vi "2P_AdapUprite_Linlin.vi"() -> ()   [LabVIEW 2015] (continued)
                                n3537 = call "waveformparamsv2.vi"("command"="add AO", "add AO"=w248) -> ()  [unwired: 3 in, 3 out]
                              }
                              frame "Matlab" {
                                w274 = 0.0 ("Repeats")
                                n3538 = local read "Meastab"() -> (w270:enum32{"X-Y Image", "Linescan", "Timetrace"})
                                n3539 = call "waveformparamsv2.vi"("command"="get") -> ("Params out"=w281:T17)  [unwired: 4 in, 2 out]
                                n3540 = Unbundle By Name(w281) -> ("AO parameters"=w278:T18)
                                n3541 = case shown="\"Timetrace\"" w270 {
                                tunnel: [w284 w285] -> w269
                                frame "X-Y Image", Default {
                                n3542 = local read "Sampling rate"() -> (w284:dbl)
                                }
                                frame "Timetrace" {
                                n3543 = local read "srateAODOtt"() -> (w285:dbl)
                                }
                                }
                                n3544 = local read "Matlab waveform path"() -> (w271:path)
                                n3545 = local read "Matlab padding value"() -> (w273:dbl)
                                n3546 = Index Array(array=w278, index=0) -> (element=w279:T19)
                                n3547 = call "matlabwfexistsdialogue.vi"("Matlab waveform path"=w271) -> ("mtalab waveform path out"=w272:path)
                                n3548 = Bundle By Name(cluster=w279, "AOtab"=2.0 ("Repeats"), "Repeats"=w274, "Cycles"=w274, "Start amplitude (V)"=w274, "Baseline (V)"=w274, "Step size (V)"=w274, "DC (%)"=w274, "Sampling frequency (Hz)"=w269, "Period (ms)"=w274, "Offset (V)"=w274, "Amplitude (V)"=w274, "Frequency"=w274, "Tri Repeats"=w274, "phase shift (ms)"=w274, "Pulses"=w274, "Matlab wave file"=w272, "padding value"=w273) -> (w276:T19)
                                n3549 = Build Array(w276) -> (w275:T18)
                                n3550 = call "waveformparamsv2.vi"("command"="add AO", "add AO"=w275) -> ()  [unwired: 3 in, 3 out]
                              }
                              frame "Triangle" {
                                w291 = 0.0 ("Offset (V)")
                                n3551 = local read "Meastab"() -> (w287:enum32{"X-Y Image", "Linescan", "Timetrace"})
                                n3552 = call "waveformparamsv2.vi"("command"="get") -> ("Params out"=w303:T17)  [unwired: 4 in, 2 out]
                                n3553 = Unbundle By Name(w303) -> ("AO parameters"=w300:T18)
                                n3554 = case shown="\"Timetrace\"" w287 {
                                tunnel: [w305 w306] -> w286
                                frame "X-Y Image", Default {
                                n3555 = local read "Sampling rate"() -> (w305:dbl)
                                }
                                frame "Timetrace" {
                                n3556 = local read "srateAODOtt"() -> (w306:dbl)
                                }
                                }
                                n3557 = local read "Tri padding value"() -> (w289:dbl)
                                n3558 = local read "Amplitude (V)"() -> (w294:dbl)
                                n3559 = local read "Tri Phase (s)"() -> (w290:dbl)
                                n3560 = local read "Tri Repeats"() -> (w292:dbl)
                                n3561 = local read "Frequency"() -> (w293:dbl)
                                n3562 = local read "Offset (V)"() -> (w295:dbl)
                                n3563 = Index Array(array=w300, index=0) -> (element=w301:T19)
                                n3564 = Bundle By Name(cluster=w301, "AOtab"=1.0 ("Repeats"), "Repeats"=w291, "Cycles"=w291, "Start amplitude (V)"=w291, "Baseline (V)"=w291, "Step size (V)"=w291, "DC (%)"=w291, "Sampling frequency (Hz)"=w286, "Period (ms)"=w291, "Offset (V)"=w295, "Amplitude (V)"=w294, "Frequency"=w293, "Tri Repeats"=w292, "phase shift (ms)"=w291, "Pulses"=w291, "Matlab wave file"=path "", "Tri phase"=w290, "padding value"=w289) -> (w298:T19)
                                n3565 = Build Array(w298) -> (w297:T18)
                                n3566 = call "waveformparamsv2.vi"("command"="add AO", "add AO"=w297) -> ()  [unwired: 3 in, 3 out]
                              }
                            }
                          }
                        }
                      }
                    }
                  }
                  frame #6 {
                    n3567 = case shown="True" w307 {
                      frame False {
                      }
                      frame True {
                        n3568 = local read "addAO"() -> (w308:bool)
                        n3569 = case shown="True" w308 {
                          frame False {
                          }
                          frame True {
                            # "add waveform to waveform array; correct waveform lengths and plot"
                            n3570 = local read "Meastab"() -> (w312:enum32{"X-Y Image", "Linescan", "Timetrace"})
                            n3571 = local read "Build analog waveform tabs"() -> (w322:enum32{"Square", "Triangle", "Matlab"})
                            n3572 = case shown="\"Timetrace\"" w312 {
                              tunnel: [w330 w331] -> w311
                              frame "X-Y Image", Default {
                                n3573 = local read "Sampling rate"() -> (w330:dbl)
                              }
                              frame "Timetrace" {
                                n3574 = local read "srateAODOtt"() -> (w331:dbl)
                              }
                            }
                            n3575 = call "waveformparamsv2.vi"("command"="get last AO") -> ("last AO"=w324:T19)  [unwired: 4 in, 2 out]
                            n3576 = case shown="\"Square\", Default" w322 {
                              tunnel: w324 -> [w334 w336 w338]
                              tunnel: [w333 w335 w337] -> w323
                              frame "Square", Default {
                                n3577 = call "generateRampedSquareWave_fromAOparameters.vi"("AO params"=w334) -> ("Waveform"=w333:waveform(dbl))  [unwired: 1 out]
                              }
                              frame "Triangle" {
                                n3578 = call "generateTriWave_fromAOparameters.vi"("AO params"=w336) -> ("Waveform"=w335:waveform(dbl))  [unwired: 1 out]
                              }
                              frame "Matlab" {
                                n3579 = call "matlabAOwffromparam.vi"("Cluster"=w338) -> ("Waveform"=w337:waveform(dbl))  [unwired: 1 out]
                              }
                            }
                            n3580 = property on="refwf" class="Ring (strict)"() -> ("RingText.Text"=w315:string)  [unwired: 2 in, 2 out]
                            n3581 = call "waveformsAObuffer.vi"("command"="get") -> ("AO wf out"=w328:waveform(dbl)[])  [unwired: 1 in]
                            n3582 = Build Array (concatenate)(w328, w323) -> (w325:waveform(dbl)[])
                            n3583 = call "waveformsDObuffer.vi"("command"="get") -> ("DO wf out"=w320:digitalwaveform[])  [unwired: 1 in]
                            n3584 = call "correctwaveformsizetemp.vi"("new sampling frequency (Hz)"=w311, "start"=FALSE, "reference waveforms to"=w315, "Analog waveforms in"=w325, "stop"=FALSE, "Digital waveforms in"=w320) -> ("analog wf out"=w318:waveform(dbl)[], "Digital wf out"=w316:digitalwaveform[], "measpoints"=w313:i32)
                            n3585 = local write "Analog Lines Plot"(w318) -> ()
                            n3586 = call "GetNumCamFramesv2.vi"("Digital Waveform Graph"=w316) -> ("Numeric"=w317:i32)  [unwired: 10 in]
                            n3587 = local write "Digital Lines Plot"(w316) -> ()
                            n3588 = call "waveformsAObuffer.vi"("AO wf in"=w318, "command"="set") -> ()  [unwired: 1 out]
                            n3589 = call "waveformsDObuffer.vi"("DO wf in"=w316, "command"="set") -> ()  [unwired: 1 out]
                            n3590 = local write "Total Camera Frames"(w317) -> ()
                            n3591 = local read "wavdet"() -> (w314:bool)
                            n3592 = case shown="True" w314 {
                              tunnel: w313 -> [_ w332]
                              frame False {
                              }
                              frame True {
                                n3593 = local write "# of frames"(w332) -> ()
                              }
                            }
                          }
                        }
                      }
                    }
                  }
                  frame #7 {
                    w340 = FALSE ("addAO")
                    # "set signaling boolean to false"
                    n3594 = case shown="True" w339 {
                      frame False {
                      }
                      frame True {
                        n3595 = local read "Build analog waveform tabs"() -> (w348:enum32{"Square", "Triangle", "Matlab"})
                        n3596 = case shown="\"Triangle\"" w348 {
                          frame "Square", Default {
                            n3597 = local write "not loaded"(FALSE ("not loaded")) -> ()
                          }
                          frame "Triangle" {
                            n3598 = local write "not loadedtri"(FALSE ("not loadedtri")) -> ()
                          }
                          frame "Matlab" {
                            n3599 = local write "not loadedml"(FALSE ("not loadedml")) -> ()
                          }
                        }
                      }
                    }
                    n3600 = local read "finite samples"() -> (w341:bool)
                    n3601 = local read "continuous"() -> (w342:bool)
                    n3602 = local read "wavdet"() -> (w343:bool)
                    n3603 = call "2pparameters.vi"("command"="get") -> ("params out"=w346:T12)  [unwired: 1 in]
                    n3604 = Bundle By Name(cluster=w346, "finite"=w341, "cont"=w342, "wavdet"=w343) -> (w344:T12)
                    n3605 = local write "addAO"(w340) -> ()
                    n3606 = property on="Add AO wave" class="Bool (strict)"("Val(Sgnl)"=w340) -> ()  [unwired: 2 in, 2 out]
                    n3607 = call "2pparameters.vi"("Params in"=w344, "command"="set") -> ()  [unwired: 1 out]
                  }
                }
              }
            }
          }
          event "AO channels": Value Change {
            n3608 = event-data() -> ()  [unwired: 1 in, 6 out]
            n3609 = local read "AO channels"() -> (w352:u32)
            n3610 = call "2pparameters.vi"("command"="get") -> ("params out"=w354:T12)  [unwired: 1 in]
            n3611 = Unbundle By Name(w354) -> ("aAO"=w353:u32[])
            n3612 = Search 1D Array(1D array=w353, element=w352) -> (index of element=w356:i32)  [unwired: 1 in]
            n3613 = Equal?(x=w356, y=-1.0) -> (x = y?=w357:bool)
            n3614 = case shown="False" w357 {
              tunnel: w356 -> [w359 _]
              frame False {
                n3615 = call "waveformparamsv2.vi"("command"="get") -> ("Params out"=w366:T17)  [unwired: 4 in, 2 out]
                n3616 = Unbundle By Name(w366) -> ("AO parameters"=w365:T18)
                n3617 = Index Array(array=w365, index=w359) -> (element=w382:T19)
                n3618 = Unbundle By Name(w382) -> ("AOtab"=w363:dbl, "Repeats"=w381:dbl, "Cycles"=w380:dbl, "Start amplitude (V)"=w379:dbl, "Baseline (V)"=w378:dbl, "Step size (V)"=w377:dbl, "DC (%)"=w376:dbl, "Sampling frequency (Hz)"=w375:dbl, "Period (ms)"=w374:dbl, "Offset (V)"=w373:dbl, "Amplitude (V)"=w372:dbl, "Frequency"=w371:dbl, "Tri Repeats"=w370:dbl, "phase shift (ms)"=w369:dbl, "Pulses"=w368:dbl, "Tri phase"=w364:dbl, "padding value"=w360:dbl, "Matlab wave file"=w361:path)
                n3619 = To Unsigned Long Integer(number=w363) -> (unsigned 32bit integer=w362:u32)
                n3620 = local write "Build analog waveform tabs"(w362) -> ()
                n3621 = local write "Matlab waveform path"(w361) -> ()
                n3622 = local write "phase shift (ms)"(w369) -> ()
                n3623 = local write "Repeats"(w381) -> ()
                n3624 = local write "Cycles"(w380) -> ()
                n3625 = local write "Amplitude (V)"(w372) -> ()
                n3626 = local write "Matlab padding value"(w360) -> ()
                n3627 = local write "Tri padding value"(w360) -> ()
                n3628 = local write "Start amplitude (V)"(w379) -> ()
                n3629 = local write "Tri Phase (s)"(w364) -> ()
                n3630 = local write "Period (ms)"(w374) -> ()
                n3631 = local write "Tri Repeats"(w370) -> ()
                n3632 = local write "Offset (V)"(w373) -> ()
                n3633 = local write "Frequency"(w371) -> ()
                n3634 = local write "Pulses"(w368) -> ()
                n3635 = local write "padding value"(w360) -> ()
                n3636 = local write "Sampling rate \ncurrent wf"(w375) -> ()
                n3637 = local write "Baseline (V)"(w378) -> ()
                n3638 = local write "Step size (V)"(w377) -> ()
                n3639 = local write "DC (%)"(w376) -> ()
              }
              frame True {
              }
            }
          }
          event "Rem AO wave": Value Change {
            n3640 = event-data() -> ("NewVal"=w383:bool)  [unwired: 1 in, 5 out]
            n3641 = case shown="True" w383 {
              frame False {
              }
              frame True {
                n3642 = stacked-sequence {
                  seq-local: [_ _ w489 _ _ _ _] -> [_ _ _ _ w509 w512 _]
                  frame #0 {
                    n3643 = local read "Measurement"() -> (w384:T4)
                    n3644 = case shown="\"Lifetime (contour)\"" w384 {
                      frame "X-Y-t movie", Default {
                        n3645 = local read "avpp"() -> (w405:i32)
                        n3646 = local read "Angle ref"() -> (w404:dbl)
                        n3647 = local read "ROI Type"() -> (w403:u16)
                        n3648 = local read "xpixels ref"() -> (w400:i32)
                        n3649 = local read "Vx-min ref"() -> (w399:dbl)
                        n3650 = local read "Vx-max ref"() -> (w398:dbl)
                        n3651 = local read "ypixels ref"() -> (w396:i32)
                        n3652 = local read "Vy-min ref"() -> (w397:dbl)
                        n3653 = local read "Vy-max ref"() -> (w393:dbl)
                        n3654 = local read "Sampling rate"() -> (w387:dbl)
                        n3655 = local read "finite samples"() -> (w388:bool)
                        n3656 = local read "continuous"() -> (w391:bool)
                        n3657 = local read "wavdet"() -> (w392:bool)
                        n3658 = local read "# of frames"() -> (w390:i32)
                        n3659 = local read "maxbufferAI"() -> (w389:i32)
                        n3660 = local read "Override AI buffer"() -> (w385:bool)
                        n3661 = call "2pparameters.vi"("command"="get") -> ("params out"=w402:T12)  [unwired: 1 in]
                        n3662 = Bundle By Name(cluster=w402, "type"="X-Y-t movie", "avpp"=w405, "Angle Img"=w404, "Xpixels Img"=w400, "Vx-min Img"=w399, "VX-max Img"=w398, "Ypixels Img"=w396, "Vy-min Img"=w397, "Vy-max Img"=w393, "srate"=w387, "srate Img"=w387, "finite"=w388, "cont"=w391, "wavdet"=w392, "measpoints"=w390, "maxbufferAI"=w389, "Drawing Mode"=w403, "Vz-reset"=0.0, "AIoverride"=w385) -> (w394:T12)
                        n3663 = call "2pparameters.vi"("Params in"=w394, "command"="set") -> ()  [unwired: 1 out]
                      }
                      frame "X-Y-Z stack" {
                        n3664 = call "2pparameters.vi"("command"="get") -> ("params out"=w409:T12)  [unwired: 1 in]
                        n3665 = Bundle By Name(cluster=w409, "type"="X-Y-Z stack") -> (w407:T12)
                        n3666 = call "2pparameters.vi"("Params in"=w407, "command"="set") -> ()  [unwired: 1 out]
                      }
                      frame "Lifetime (scan)" {
                        n3667 = call "2pparameters.vi"("command"="get") -> ("params out"=w414:T12)  [unwired: 1 in]
                        n3668 = Bundle By Name(cluster=w414, "type"="Lifetime (scan)") -> (w412:T12)
                        n3669 = call "2pparameters.vi"("Params in"=w412, "command"="set") -> ()  [unwired: 1 out]
                      }
                      frame "Lifetime (contour)" {
                        n3670 = local read "Vy-min draw"() -> (w424:dbl)
                        n3671 = local read "Vy-max draw"() -> (w423:dbl)
                        n3672 = local read "Vx-min draw"() -> (w426:dbl)
                        n3673 = local read "Vx-max draw"() -> (w425:dbl)
                        n3674 = local read "xpixels ref"() -> (w422:i32)
                        n3675 = local read "ypixels ref"() -> (w421:i32)
                        n3676 = local read "ROI Type"() -> (w420:u16)
                        n3677 = local read "srateAODOtt"() -> (w431:dbl)
                        n3678 = local read "# of frames"() -> (w436:i32)
                        n3679 = local read "refreshtime"() -> (w428:dbl)
                        n3680 = local read "Pel"() -> (w419:dbl)
                        n3681 = local read "bin"() -> (w434:dbl)
                        n3682 = local read "Override AI buffer"() -> (w417:bool)
                        n3683 = local read "finite samples"() -> (w443:bool)
                        n3684 = local read "srateAODOtt"() -> (w430:dbl)
                        n3685 = local read "srateAODOtt"() -> (w437:dbl)
                        n3686 = local read "continuous"() -> (w442:bool)
                        n3687 = local read "Angle ref"() -> (w427:dbl)
                        n3688 = local read "wavdet"() -> (w444:bool)
                        n3689 = local read "Vx-ref"() -> (w439:dbl)
                        n3690 = local read "Vy-ref"() -> (w441:dbl)
                        n3691 = local read "avpp"() -> (w440:i32)
                        n3692 = call "tt_timeandsamples.vi"("bin"=w434, "refreshtime"=w428, "srateAODOtt"=w431, "tot#ofsamples"=w436) -> ("refreshrate"=w432:dbl, "refreshbuffer"=w433:i32, "timetracecycles"=w438:i32)  [unwired: 5 in]
                        n3693 = local read "bin"() -> (w435:dbl)
                        n3694 = call "2pparameters.vi"("command"="get") -> ("params out"=w447:T12)  [unwired: 1 in]
                        n3695 = Bundle By Name(cluster=w447, "Drawing Mode"=w420, "measpoints"=w436, "tt_cycles"=w438, "refreshbuffer"=w433, "refreshrate"=w432, "Vx-ref"=w439, "Vy-ref"=w441, "srate"=w430, "finite"=w443, "cont"=w442, "wavdet"=w444, "avpp"=w440, "srateAODO"=w437, "bufferAI"=w433, "bin"=w435, "Angle Img"=w427, "Vxminref"=w426, "Vxmaxref"=w425, "Vyminref"=w424, "Vymaxref"=w423, "Xpixels Img"=w422, "Ypixels Img"=w421, "Pel"=w419, "Vz-reset"=0.0, "AIoverride"=w417, "type"="Lifetime (contour)") -> (w445:T12)
                        n3696 = Reciprocal(x=w432) -> (1/x=w429:dbl)
                        n3697 = local write "refreshtime"(w429) -> ()
                        n3698 = call "2pparameters.vi"("Params in"=w445, "command"="set") -> ()  [unwired: 1 out]
                      }
                      frame "X-Y-Z-t movie" {
                      }
                      frame "linescan" {
                      }
                      frame "Timetrace" {
                        n3699 = local read "Vy-min draw"() -> (w457:dbl)
                        n3700 = local read "Vy-max draw"() -> (w456:dbl)
                        n3701 = local read "Vx-min draw"() -> (w459:dbl)
                        n3702 = local read "Vx-max draw"() -> (w458:dbl)
                        n3703 = local read "xpixels ref"() -> (w455:i32)
                        n3704 = local read "ypixels ref"() -> (w454:i32)
                        n3705 = local read "ROI Type"() -> (w453:u16)
                        n3706 = local read "srateAODOtt"() -> (w464:dbl)
                        n3707 = local read "# of frames"() -> (w469:i32)
                        n3708 = local read "refreshtime"() -> (w461:dbl)
                        n3709 = local read "Pel"() -> (w452:dbl)
                        n3710 = local read "bin"() -> (w467:dbl)
                        n3711 = local read "Override AI buffer"() -> (w450:bool)
                        n3712 = local read "finite samples"() -> (w476:bool)
                        n3713 = local read "srateAODOtt"() -> (w463:dbl)
                        n3714 = local read "srateAODOtt"() -> (w470:dbl)
                        n3715 = local read "continuous"() -> (w475:bool)
                        n3716 = local read "Angle ref"() -> (w460:dbl)
                        n3717 = local read "wavdet"() -> (w477:bool)
                        n3718 = local read "Vx-ref"() -> (w472:dbl)
                        n3719 = local read "Vy-ref"() -> (w474:dbl)
                        n3720 = local read "avpp"() -> (w473:i32)
                        n3721 = call "tt_timeandsamples.vi"("bin"=w467, "refreshtime"=w461, "srateAODOtt"=w464, "tot#ofsamples"=w469) -> ("refreshrate"=w465:dbl, "refreshbuffer"=w466:i32, "timetracecycles"=w471:i32)  [unwired: 5 in]
                        n3722 = local read "bin"() -> (w468:dbl)
                        n3723 = call "2pparameters.vi"("command"="get") -> ("params out"=w480:T12)  [unwired: 1 in]
                        n3724 = Bundle By Name(cluster=w480, "Drawing Mode"=w453, "measpoints"=w469, "tt_cycles"=w471, "refreshbuffer"=w466, "refreshrate"=w465, "Vx-ref"=w472, "Vy-ref"=w474, "srate"=w463, "finite"=w476, "cont"=w475, "wavdet"=w477, "avpp"=w473, "srateAODO"=w470, "bufferAI"=w466, "bin"=w468, "Angle Img"=w460, "Vxminref"=w459, "Vxmaxref"=w458, "Vyminref"=w457, "Vymaxref"=w456, "Xpixels Img"=w455, "Ypixels Img"=w454, "Pel"=w452, "Vz-reset"=0.0, "AIoverride"=w450, "type"="Timetrace") -> (w478:T12)
                        n3725 = Reciprocal(x=w465) -> (1/x=w462:dbl)
                        n3726 = local write "refreshtime"(w462) -> ()
                        n3727 = call "2pparameters.vi"("Params in"=w478, "command"="set") -> ()  [unwired: 1 out]
                      }
                      frame "Lifetime (point)" {
                      }
                    }
                  }
                  frame #1 {
                    w483 = FALSE ("wavdet")
                    n3728 = call "2pparameters.vi"("command"="get") -> ("params out"=w487:T12)  [unwired: 1 in]
                    n3729 = Bundle By Name(cluster=w487, "finite"=w483, "cont"=w483, "wavdet"=TRUE) -> (w484:T12)
                    n3730 = call "2pparameters.vi"("Params in"=w484, "command"="set") -> ()  [unwired: 1 out]
                  }
                  frame #2 {
                    # "remove channel from numbers array"
                    n3731 = local read "AO channels"() -> (w494:u32)
                    n3732 = call "2pparameters.vi"("command"="get") -> ("params out"=w492:T12)  [unwired: 1 in]
                    n3733 = in-place {
                      in-place-border: w494 -> [w500]
                      in-place-border: [w497] -> w495
                      in-place-border: [w496] -> w489
                      n3734 = in-place-cluster #49(w492) -> ("aAO"=w499:u32[])
                      n3735 = call "remove channel from active arrayv2.vi"("line array in"=w499, "line to remove"=w500) -> ("line array out"=w498:u32[], "removal"=w497:bool, "index"=w496:i32)
                      n3736 = in-place-cluster #49("aAO"=w498) -> (w490:T12)
                    }
                    n3737 = local write "remAO"(w495) -> ()
                    n3738 = call "2pparameters.vi"("Params in"=w490, "command"="set") -> ()  [unwired: 1 out]
                  }
                  frame #3 {
                    n3739 = local read "remAO"() -> (w501:bool)
                    n3740 = case shown="True" w501 {
                      frame False {
                      }
                      frame True {
                        n3741 = call "Used AO lines.vi"() -> ("used AO names"=w505:string[], "used AO lines"=w507:tag[])  [unwired: 2 in]
                        n3742 = control-ref of="Analog Lines Plot"() -> (w506:refnum<vi>)
                        n3743 = control-ref of="Digital Lines Plot"() -> (w504:refnum<vi>)
                        n3744 = call "Used DO lines.vi"() -> ("used DO names"=w503:string[], "used DO lines"=w502:tag[])  [unwired: 2 in]
                        n3745 = local write "Analog Used Lines"(w507) -> ()
                        n3746 = local write "Analog Used Names"(w505) -> ()
                        n3747 = local write "Digital Used Lines"(w502) -> ()
                        n3748 = local write "Digital Used Names"(w503) -> ()
                        n3749 = call "prepDOWaveplot.vi"("DigitalGraph in"=w504, "used DO names"=w503) -> ()  [unwired: 1 in]
                        n3750 = call "prepAOWaveplot.vi"("WaveformGraph in"=w506, "Analog Used Names"=w505) -> ()  [unwired: 1 in]
                      }
                    }
                  }
                  frame #4 {
                    n3751 = local read "remAO"() -> (w508:bool)
                    n3752 = case shown="True" w508 {
                      tunnel: w509 -> [_ w510]
                      frame False {
                      }
                      frame True {
                        n3753 = call "waveformparamsv2.vi"("command"="rem AO", "index"=w510) -> ()  [unwired: 3 in, 3 out]
                      }
                    }
                  }
                  frame #5 {
                    n3754 = local read "remAO"() -> (w513:bool)
                    n3755 = case shown="True" w513 {
                      tunnel: w512 -> [_ w532]
                      frame False {
                      }
                      frame True {
                        n3756 = local read "Meastab"() -> (w517:enum32{"X-Y Image", "Linescan", "Timetrace"})
                        n3757 = property on="refwf" class="Ring (strict)"() -> ("RingText.Text"=w520:string)  [unwired: 2 in, 2 out]
                        n3758 = case shown="\"Timetrace\"" w517 {
                          tunnel: [w533 w534] -> w516
                          frame "X-Y Image", Default {
                            n3759 = local read "Sampling rate"() -> (w533:dbl)
                          }
                          frame "Timetrace" {
                            n3760 = local read "srateAODOtt"() -> (w534:dbl)
                          }
                        }
                        n3761 = call "waveformsAObuffer.vi"("command"="get") -> ("AO wf out"=w529:waveform(dbl)[])  [unwired: 1 in]
                        n3762 = call "waveformsDObuffer.vi"("command"="get") -> ("DO wf out"=w526:digitalwaveform[])  [unwired: 1 in]
                        n3763 = Delete From Array(array=w529, length=1, index=w532) -> (array with subset deleted=w521:waveform(dbl)[])  [unwired: 1 out]
                        n3764 = call "correctwaveformsizetemp.vi"("new sampling frequency (Hz)"=w516, "start"=FALSE, "reference waveforms to"=w520, "Analog waveforms in"=w521, "stop"=FALSE, "Digital waveforms in"=w526) -> ("analog wf out"=w524:waveform(dbl)[], "Digital wf out"=w522:digitalwaveform[], "measpoints"=w518:i32)
                        n3765 = local write "Analog Lines Plot"(w524) -> ()
                        n3766 = call "GetNumCamFramesv2.vi"("Digital Waveform Graph"=w522) -> ("Numeric"=w523:i32)  [unwired: 10 in]
                        n3767 = local write "Digital Lines Plot"(w522) -> ()
                        n3768 = call "waveformsAObuffer.vi"("AO wf in"=w524, "command"="set") -> ()  [unwired: 1 out]
                        n3769 = call "waveformsDObuffer.vi"("DO wf in"=w522, "command"="set") -> ()  [unwired: 1 out]
                        n3770 = local read "wavdet"() -> (w519:bool)
                        n3771 = local write "Total Camera Frames"(w523) -> ()
                        n3772 = case shown="True" w519 {
                          tunnel: w518 -> [_ w535]
                          frame False {
                          }
                          frame True {
                            n3773 = local write "# of frames"(w535) -> ()
                          }
                        }
                      }
                    }
                  }
                  frame #6 {
                    w536 = FALSE ("remAO")
                    n3774 = local read "finite samples"() -> (w537:bool)
                    n3775 = local read "continuous"() -> (w538:bool)
                    n3776 = local read "wavdet"() -> (w539:bool)
                    n3777 = call "2pparameters.vi"("command"="get") -> ("params out"=w542:T12)  [unwired: 1 in]
                    n3778 = Bundle By Name(cluster=w542, "finite"=w537, "cont"=w538, "wavdet"=w539) -> (w540:T12)
                    n3779 = local write "remAO"(w536) -> ()
                    n3780 = property on="Rem AO wave" class="Bool (strict)"("Val(Sgnl)"=w536) -> ()  [unwired: 2 in, 2 out]
                    n3781 = call "2pparameters.vi"("Params in"=w540, "command"="set") -> ()  [unwired: 1 out]
                  }
                }
              }
            }
          }
          event "Add DO wave": Value Change {
            n3782 = event-data() -> ("NewVal"=w544:bool)  [unwired: 1 in, 5 out]
            n3783 = case shown="True" w544 {
              frame False {
              }
              frame True {
                n3784 = stacked-sequence {
                  seq-local: [_ _ _ _ _ w704 _ _] -> [_ _ _ _ _ _ w719 _]
                  frame #0 {
                    n3785 = local read "Measurement"() -> (w545:T4)
                    n3786 = case shown="\"X-Y-t movie\", Default" w545 {
                      frame "X-Y-t movie", Default {
                        n3787 = local read "avpp"() -> (w566:i32)
                        n3788 = local read "Angle ref"() -> (w565:dbl)
                        n3789 = local read "ROI Type"() -> (w564:u16)
                        n3790 = local read "xpixels ref"() -> (w561:i32)
                        n3791 = local read "Vx-min ref"() -> (w560:dbl)
                        n3792 = local read "Vx-max ref"() -> (w559:dbl)
                        n3793 = local read "ypixels ref"() -> (w557:i32)
                        n3794 = local read "Vy-min ref"() -> (w558:dbl)
                        n3795 = local read "Vy-max ref"() -> (w554:dbl)
                        n3796 = local read "Sampling rate"() -> (w548:dbl)
                        n3797 = local read "finite samples"() -> (w549:bool)
                        n3798 = local read "continuous"() -> (w552:bool)
                        n3799 = local read "wavdet"() -> (w553:bool)
                        n3800 = local read "# of frames"() -> (w551:i32)
                        n3801 = local read "maxbufferAI"() -> (w550:i32)
                        n3802 = local read "Override AI buffer"() -> (w546:bool)
                        n3803 = call "2pparameters.vi"("command"="get") -> ("params out"=w563:T12)  [unwired: 1 in]
                        n3804 = Bundle By Name(cluster=w563, "type"="X-Y-t movie", "avpp"=w566, "Angle Img"=w565, "Xpixels Img"=w561, "Vx-min Img"=w560, "VX-max Img"=w559, "Ypixels Img"=w557, "Vy-min Img"=w558, "Vy-max Img"=w554, "srate"=w548, "srate Img"=w548, "finite"=w549, "cont"=w552, "wavdet"=w553, "measpoints"=w551, "maxbufferAI"=w550, "Drawing Mode"=w564, "Vz-reset"=0.0, "AIoverride"=w546) -> (w555:T12)
                        n3805 = call "2pparameters.vi"("Params in"=w555, "command"="set") -> ()  [unwired: 1 out]
                      }
                      frame "X-Y-Z stack" {
                        n3806 = call "2pparameters.vi"("command"="get") -> ("params out"=w570:T12)  [unwired: 1 in]
                        n3807 = Bundle By Name(cluster=w570, "type"="X-Y-Z stack") -> (w568:T12)
                        n3808 = call "2pparameters.vi"("Params in"=w568, "command"="set") -> ()  [unwired: 1 out]
                      }
                      frame "Lifetime (scan)" {
                        n3809 = call "2pparameters.vi"("command"="get") -> ("params out"=w575:T12)  [unwired: 1 in]
                        n3810 = Bundle By Name(cluster=w575, "type"="Lifetime (scan)") -> (w573:T12)
                        n3811 = call "2pparameters.vi"("Params in"=w573, "command"="set") -> ()  [unwired: 1 out]
                      }
                      frame "Lifetime (contour)" {
                        n3812 = local read "Vy-min draw"() -> (w585:dbl)
                        n3813 = local read "Vy-max draw"() -> (w584:dbl)
                        n3814 = local read "Vx-min draw"() -> (w587:dbl)
                        n3815 = local read "Vx-max draw"() -> (w586:dbl)
                        n3816 = local read "xpixels ref"() -> (w583:i32)
                        n3817 = local read "ypixels ref"() -> (w582:i32)
                        n3818 = local read "ROI Type"() -> (w581:u16)
                        n3819 = local read "srateAODOtt"() -> (w592:dbl)
                        n3820 = local read "# of frames"() -> (w597:i32)
                        n3821 = local read "refreshtime"() -> (w589:dbl)
                        n3822 = local read "Pel"() -> (w580:dbl)
                        n3823 = local read "bin"() -> (w595:dbl)
                        n3824 = local read "Override AI buffer"() -> (w578:bool)
                        n3825 = local read "finite samples"() -> (w604:bool)
                        n3826 = local read "srateAODOtt"() -> (w591:dbl)
                        n3827 = local read "srateAODOtt"() -> (w598:dbl)
                        n3828 = local read "continuous"() -> (w603:bool)
                        n3829 = local read "Angle ref"() -> (w588:dbl)
                        n3830 = local read "wavdet"() -> (w605:bool)
                        n3831 = local read "Vx-ref"() -> (w600:dbl)
                        n3832 = local read "Vy-ref"() -> (w602:dbl)
                        n3833 = local read "avpp"() -> (w601:i32)
                        n3834 = call "tt_timeandsamples.vi"("bin"=w595, "refreshtime"=w589, "srateAODOtt"=w592, "tot#ofsamples"=w597) -> ("refreshrate"=w593:dbl, "refreshbuffer"=w594:i32, "timetracecycles"=w599:i32)  [unwired: 5 in]
                        n3835 = local read "bin"() -> (w596:dbl)
                        n3836 = call "2pparameters.vi"("command"="get") -> ("params out"=w608:T12)  [unwired: 1 in]
                        n3837 = Bundle By Name(cluster=w608, "Drawing Mode"=w581, "measpoints"=w597, "tt_cycles"=w599, "refreshbuffer"=w594, "refreshrate"=w593, "Vx-ref"=w600, "Vy-ref"=w602, "srate"=w591, "finite"=w604, "cont"=w603, "wavdet"=w605, "avpp"=w601, "srateAODO"=w598, "bufferAI"=w594, "bin"=w596, "Angle Img"=w588, "Vxminref"=w587, "Vxmaxref"=w586, "Vyminref"=w585, "Vymaxref"=w584, "Xpixels Img"=w583, "Ypixels Img"=w582, "Pel"=w580, "Vz-reset"=0.0, "AIoverride"=w578, "type"="Lifetime (contour)") -> (w606:T12)
                        n3838 = Reciprocal(x=w593) -> (1/x=w590:dbl)
                        n3839 = local write "refreshtime"(w590) -> ()
                        n3840 = call "2pparameters.vi"("Params in"=w606, "command"="set") -> ()  [unwired: 1 out]
                      }
                      frame "X-Y-Z-t movie" {
                      }
                      frame "linescan" {
                      }
                      frame "Timetrace" {
                        n3841 = local read "Vy-min draw"() -> (w618:dbl)
                        n3842 = local read "Vy-max draw"() -> (w617:dbl)
                        n3843 = local read "Vx-min draw"() -> (w620:dbl)
                        n3844 = local read "Vx-max draw"() -> (w619:dbl)
                        n3845 = local read "xpixels ref"() -> (w616:i32)
                        n3846 = local read "ypixels ref"() -> (w615:i32)
                        n3847 = local read "ROI Type"() -> (w614:u16)
                        n3848 = local read "srateAODOtt"() -> (w625:dbl)
                        n3849 = local read "# of frames"() -> (w630:i32)
                        n3850 = local read "refreshtime"() -> (w622:dbl)
                        n3851 = local read "Pel"() -> (w613:dbl)
                        n3852 = local read "bin"() -> (w628:dbl)
                        n3853 = local read "Override AI buffer"() -> (w611:bool)
                        n3854 = local read "finite samples"() -> (w637:bool)
                        n3855 = local read "srateAODOtt"() -> (w624:dbl)
                        n3856 = local read "srateAODOtt"() -> (w631:dbl)
                        n3857 = local read "continuous"() -> (w636:bool)
                        n3858 = local read "Angle ref"() -> (w621:dbl)
                        n3859 = local read "wavdet"() -> (w638:bool)
                        n3860 = local read "Vx-ref"() -> (w633:dbl)
                        n3861 = local read "Vy-ref"() -> (w635:dbl)
                        n3862 = local read "avpp"() -> (w634:i32)
                        n3863 = call "tt_timeandsamples.vi"("bin"=w628, "refreshtime"=w622, "srateAODOtt"=w625, "tot#ofsamples"=w630) -> ("refreshrate"=w626:dbl, "refreshbuffer"=w627:i32, "timetracecycles"=w632:i32)  [unwired: 5 in]
                        n3864 = local read "bin"() -> (w629:dbl)
                        n3865 = call "2pparameters.vi"("command"="get") -> ("params out"=w641:T12)  [unwired: 1 in]
                        n3866 = Bundle By Name(cluster=w641, "Drawing Mode"=w614, "measpoints"=w630, "tt_cycles"=w632, "refreshbuffer"=w627, "refreshrate"=w626, "Vx-ref"=w633, "Vy-ref"=w635, "srate"=w624, "finite"=w637, "cont"=w636, "wavdet"=w638, "avpp"=w634, "srateAODO"=w631, "bufferAI"=w627, "bin"=w629, "Angle Img"=w621, "Vxminref"=w620, "Vxmaxref"=w619, "Vyminref"=w618, "Vymaxref"=w617, "Xpixels Img"=w616, "Ypixels Img"=w615, "Pel"=w613, "Vz-reset"=0.0, "AIoverride"=w611, "type"="Timetrace") -> (w639:T12)
                        n3867 = Reciprocal(x=w626) -> (1/x=w623:dbl)
                        n3868 = local write "refreshtime"(w623) -> ()
                        n3869 = call "2pparameters.vi"("Params in"=w639, "command"="set") -> ()  [unwired: 1 out]
                      }
                      frame "Lifetime (point)" {
                      }
                    }
                  }
                  frame #1 {
                    w644 = FALSE ("wavdet")
                    n3870 = call "2pparameters.vi"("command"="get") -> ("params out"=w648:T12)  [unwired: 1 in]
                    n3871 = Bundle By Name(cluster=w648, "finite"=w644, "cont"=w644, "wavdet"=TRUE) -> (w645:T12)
                    n3872 = call "2pparameters.vi"("Params in"=w645, "command"="set") -> ()  [unwired: 1 out]
                  }
                  frame #2 {
                    n3873 = local read "DO channels"() -> (w655:u16)
                    n3874 = call "2pparameters.vi"("command"="get") -> ("params out"=w653:T12)  [unwired: 1 in]
                    n3875 = in-place {
                      in-place-border: w655 -> [w659]
                      in-place-border: [w656] -> w650
                      n3876 = in-place-cluster #50(w653) -> ("aDO"=w658:u32[])
                      n3877 = call "add channel to active arrayv2.vi"("line array in"=w658, "line to add"=w659) -> ("line array out"=w657:u32[], "addition"=w656:bool)  [unwired: 1 out]
                      n3878 = in-place-cluster #50("aDO"=w657) -> (w651:T12)
                    }
                    n3879 = local write "addDO"(w650) -> ()
                    n3880 = call "2pparameters.vi"("Params in"=w651, "command"="set") -> ()  [unwired: 1 out]
                  }
                  frame #3 {
                    n3881 = local read "addDO"() -> (w660:bool)
                    n3882 = case shown="True" w660 {
                      frame False {
                      }
                      frame True {
                        n3883 = call "Used AO lines.vi"() -> ("used AO names"=w664:string[], "used AO lines"=w666:tag[])  [unwired: 2 in]
                        n3884 = control-ref of="Analog Lines Plot"() -> (w665:refnum<vi>)
                        n3885 = control-ref of="Digital Lines Plot"() -> (w663:refnum<vi>)
                        n3886 = call "Used DO lines.vi"() -> ("used DO names"=w662:string[], "used DO lines"=w661:tag[])  [unwired: 2 in]
                        n3887 = local write "Analog Used Lines"(w666) -> ()
                        n3888 = local write "Analog Used Names"(w664) -> ()
                        n3889 = local write "Digital Used Lines"(w661) -> ()
                        n3890 = local write "Digital Used Names"(w662) -> ()
                        n3891 = call "prepDOWaveplot.vi"("DigitalGraph in"=w663, "used DO names"=w662) -> ()  [unwired: 1 in]
                        n3892 = call "prepAOWaveplot.vi"("WaveformGraph in"=w665, "Analog Used Names"=w664) -> ()  [unwired: 1 in]
                      }
                    }
                  }
                  frame #4 {
                    n3893 = local read "addDO"() -> (w667:bool)
                    n3894 = case shown="True" w667 {
                      frame False {
                      }
                      frame True {
                        n3895 = local read "Build digital waveform tabs"() -> (w668:enum32{"Simple", "Matlab"})
                        n3896 = case shown="\"Matlab\"" w668 {
                          frame "Simple", Default {
                            n3897 = local read "Meastab"() -> (w670:enum32{"X-Y Image", "Linescan", "Timetrace"})
                            n3898 = call "waveformparamsv2.vi"("command"="get") -> ("Params out"=w684:T17)  [unwired: 4 in, 2 out]
                            n3899 = case shown="\"Timetrace\"" w670 {
                              tunnel: [w686 w687] -> w669
                              frame "X-Y Image", Default {
                                n3900 = local read "Sampling rate"() -> (w686:dbl)
                              }
                              frame "Timetrace" {
                                n3901 = local read "srateAODOtt"() -> (w687:dbl)
                              }
                            }
                            n3902 = Unbundle By Name(w684) -> ("DO parameters"=w682:T20)
                            n3903 = local read "Digital padding value"() -> (w673:dbl)
                            n3904 = local read "Digital time offset (s)"() -> (w674:dbl)
                            n3905 = local read "Digital phase (s)"() -> (w676:dbl)
                            n3906 = local read "Digital Freq (Hz)"() -> (w675:dbl)
                            n3907 = local read "Digital DC (%)"() -> (w677:dbl)
                            n3908 = Index Array(array=w682, index=0) -> (element=w681:T21)
                            n3909 = Bundle By Name(cluster=w681, "Digital DC (%)"=w677, "Digital phase"=w676, "Digital Freq (Hz)"=w675, "Sampling frequency (Hz)"=w669, "Digital time offset (s)"=w674, "padding value"=w673, "matlab wave file"=path "", "DOtab"=0.0) -> (w679:T21)
                            n3910 = Build Array(w679) -> (w678:T20)
                            n3911 = call "waveformparamsv2.vi"("command"="add DO", "add DO"=w678) -> ()  [unwired: 3 in, 3 out]
                          }
                          frame "Matlab" {
                            w691 = 0.0 ("DOtab")
                            n3912 = local read "Meastab"() -> (w689:enum32{"X-Y Image", "Linescan", "Timetrace"})
                            n3913 = call "waveformparamsv2.vi"("command"="get") -> ("Params out"=w700:T17)  [unwired: 4 in, 2 out]
                            n3914 = case shown="\"Timetrace\"" w689 {
                              tunnel: [w702 w703] -> w688
                              frame "X-Y Image", Default {
                                n3915 = local read "Sampling rate"() -> (w702:dbl)
                              }
                              frame "Timetrace" {
                                n3916 = local read "srateAODOtt"() -> (w703:dbl)
                              }
                            }
                            n3917 = Unbundle By Name(w700) -> ("DO parameters"=w698:T20)
                            n3918 = local read "Matlab waveform path DO"() -> (w690:path)
                            n3919 = local read "Matlab padding value DO"() -> (w693:dbl)
                            n3920 = Index Array(array=w698, index=0) -> (element=w697:T21)
                            n3921 = Bundle By Name(cluster=w697, "Digital DC (%)"=w691, "Digital phase"=w691, "Digital Freq (Hz)"=w691, "Sampling frequency (Hz)"=w688, "Digital time offset (s)"=w691, "padding value"=w693, "matlab wave file"=w690, "DOtab"=1.0) -> (w695:T21)
                            n3922 = Build Array(w695) -> (w694:T20)
                            n3923 = call "waveformparamsv2.vi"("command"="add DO", "add DO"=w694) -> ()  [unwired: 3 in, 3 out]
                          }
                        }
                      }
                    }
                  }
                  frame #5 {
                    n3924 = local read "addDO"() -> (w705:bool)
                    n3925 = case shown="True" w705 {
                      tunnel: [_ w706] -> w704
                      frame False {
                      }
                      frame True {
                        n3926 = property on="refwf" class="Ring (strict)"() -> ("RingText.Text"=w711:string)  [unwired: 2 in, 2 out]
                        n3927 = call "waveformsDObuffer.vi"("command"="get") -> ("DO wf out"=w710:digitalwaveform[])  [unwired: 1 in]
                        n3928 = call "waveformsAObuffer.vi"("command"="get") -> ("AO wf out"=w708:waveform(dbl)[])  [unwired: 1 in]
                        n3929 = call "referfencesize.vi"("Digital waveforms in"=w710, "Analog waveforms in"=w708, "reference waveforms to"=w711) -> ("number of samples"=w706:i32)  [unwired: 2 in]
                      }
                    }
                  }
                  frame #6 {
                    n3930 = local read "Build digital waveform tabs"() -> (w722:enum32{"Simple", "Matlab"})
                    n3931 = call "waveformparamsv2.vi"("command"="get last DO") -> ("last DO"=w721:T21)  [unwired: 4 in, 2 out]
                    n3932 = local read "Meastab"() -> (w715:enum32{"X-Y Image", "Linescan", "Timetrace"})
                    n3933 = call "waveformsDObuffer.vi"("command"="get") -> ("DO wf out"=w720:digitalwaveform[])  [unwired: 1 in]
                    n3934 = case shown="\"Simple\", Default" w722 {
                      tunnel: w721 -> [w739 w741]
                      tunnel: w719 -> [w738 _]
                      tunnel: [w737 w740] -> w718
                      frame "Simple", Default {
                        n3935 = call "simple digital from wf params.vi"("waveform params"=w739, "number of samples"=w738) -> ("digital waveform"=w737:digitalwaveform)
                      }
                      frame "Matlab" {
                        n3936 = call "matlabDOwffromparam.vi"("waveform params"=w741) -> ("digital waveform"=w740:digitalwaveform)
                      }
                    }
                    n3937 = property on="refwf" class="Ring (strict)"() -> ("RingText.Text"=w725:string)  [unwired: 2 in, 2 out]
                    n3938 = case shown="\"Timetrace\"" w715 {
                      tunnel: [w734 w735] -> w714
                      frame "X-Y Image", Default {
                        n3939 = local read "Sampling rate"() -> (w734:dbl)
                      }
                      frame "Timetrace" {
                        n3940 = local read "srateAODOtt"() -> (w735:dbl)
                      }
                    }
                    n3941 = call "waveformsAObuffer.vi"("command"="get") -> ("AO wf out"=w733:waveform(dbl)[])  [unwired: 1 in]
                    n3942 = Build Array (concatenate)(w720, w718) -> (w724:digitalwaveform[])
                    n3943 = call "correctwaveformsizetemp.vi"("new sampling frequency (Hz)"=w714, "start"=FALSE, "reference waveforms to"=w725, "Analog waveforms in"=w733, "stop"=FALSE, "Digital waveforms in"=w724) -> ("analog wf out"=w728:waveform(dbl)[], "Digital wf out"=w726:digitalwaveform[], "measpoints"=w716:i32)
                    n3944 = local write "Analog Lines Plot"(w728) -> ()
                    n3945 = call "GetNumCamFramesv2.vi"("Digital Waveform Graph"=w726) -> ("Numeric"=w727:i32)  [unwired: 10 in]
                    n3946 = local write "Digital Lines Plot"(w726) -> ()
                    n3947 = call "waveformsAObuffer.vi"("AO wf in"=w728, "command"="set") -> ()  [unwired: 1 out]
                    n3948 = call "waveformsDObuffer.vi"("DO wf in"=w726, "command"="set") -> ()  [unwired: 1 out]
                    n3949 = local write "Total Camera Frames"(w727) -> ()
                    n3950 = local read "wavdet"() -> (w717:bool)
                    n3951 = case shown="True" w717 {
                      tunnel: w716 -> [_ w736]
                      frame False {
                      }
                      frame True {
                        n3952 = local write "# of frames"(w736) -> ()
                      }
                    }
                  }
                  frame #7 {
                    w743 = FALSE ("addAO")
                    n3953 = local read "Build digital waveform tabs"() -> (w742:enum32{"Simple", "Matlab"})
                    n3954 = case shown="\"Simple\", Default" w742 {
                      frame "Simple", Default {
                        n3955 = local write "not loadedDO"(FALSE ("not loadedDO")) -> ()
                      }
                      frame "Matlab" {
                        n3956 = local write "not loadedDOml"(FALSE ("not loadedDO")) -> ()
                      }
                    }
                    n3957 = local read "finite samples"() -> (w744:bool)
                    n3958 = local read "continuous"() -> (w745:bool)
                    n3959 = local read "wavdet"() -> (w746:bool)
                    n3960 = call "2pparameters.vi"("command"="get") -> ("params out"=w749:T12)  [unwired: 1 in]
                    n3961 = Bundle By Name(cluster=w749, "finite"=w744, "cont"=w745, "wavdet"=w746) -> (w747:T12)
                    n3962 = call "2pparameters.vi"("Params in"=w747, "command"="set") -> ()  [unwired: 1 out]
                    n3963 = local write "addDO"(w743) -> ()
                    n3964 = property on="Add DO wave" class="Bool (strict)"("Val(Sgnl)"=w743) -> ()  [unwired: 2 in, 2 out]
                  }
                }
              }
            }
          }
          event "DO channels": Value Change {
            n3965 = event-data() -> ()  [unwired: 1 in, 6 out]
            n3966 = local read "DO channels"() -> (w755:u16)
            n3967 = call "2pparameters.vi"("command"="get") -> ("params out"=w757:T12)  [unwired: 1 in]
            n3968 = Unbundle By Name(w757) -> ("aDO"=w756:u32[])
            n3969 = Search 1D Array(1D array=w756, element=w755) -> (index of element=w754:i32)  [unwired: 1 in]
            n3970 = Equal?(x=w754, y=-1.0) -> (x = y?=w753:bool)
            n3971 = case shown="False" w753 {
              tunnel: w754 -> [w772 _]
              frame False {
                n3972 = call "waveformparamsv2.vi"("command"="get") -> ("Params out"=w767:T17)  [unwired: 4 in, 2 out]
                n3973 = Unbundle By Name(w767) -> ("DO parameters"=w765:T20)
                n3974 = Index Array(array=w765, index=w772) -> (element=w771:T21)
                n3975 = Unbundle By Name(w771) -> ("Digital DC (%)"=w770:dbl, "Digital phase"=w769:dbl, "Digital Freq (Hz)"=w768:dbl, "Sampling frequency (Hz)"=w760:dbl, "Digital time offset (s)"=w764:dbl, "padding value"=w763:dbl, "matlab wave file"=w762:path, "DOtab"=w761:dbl)
                n3976 = local write "Build digital waveform tabs"(w761) -> ()
                n3977 = local write "Digital DC (%)"(w770) -> ()
                n3978 = local write "Matlab waveform path DO"(w762) -> ()
                n3979 = local write "Digital time offset (s)"(w764) -> ()
                n3980 = local write "Matlab padding value DO"(w763) -> ()
                n3981 = local write "Digital padding value"(w763) -> ()
                n3982 = local write "Sampling rate \ncurrent wf"(w760) -> ()
                n3983 = local write "Digital Freq (Hz)"(w768) -> ()
                n3984 = local write "Digital phase (s)"(w769) -> ()
              }
              frame True {
              }
            }
          }
          event "Rem DO wave": Value Change {
            n3985 = event-data() -> ("NewVal"=w773:bool)  [unwired: 1 in, 5 out]
            n3986 = case shown="True" w773 {
              frame False {
              }
              frame True {
                n3987 = stacked-sequence {
                  seq-local: [_ _ w879 _ _ _ _] -> [_ _ _ _ w898 w909 _]
                  frame #0 {
                    n3988 = local read "Measurement"() -> (w774:T4)
                    n3989 = case shown="\"linescan\"" w774 {
                      frame "X-Y-t movie", Default {
                        n3990 = local read "avpp"() -> (w795:i32)
                        n3991 = local read "Angle ref"() -> (w794:dbl)
                        n3992 = local read "ROI Type"() -> (w793:u16)
                        n3993 = local read "xpixels ref"() -> (w790:i32)
                        n3994 = local read "Vx-min ref"() -> (w789:dbl)
                        n3995 = local read "Vx-max ref"() -> (w788:dbl)
                        n3996 = local read "ypixels ref"() -> (w786:i32)
                        n3997 = local read "Vy-min ref"() -> (w787:dbl)
                        n3998 = local read "Vy-max ref"() -> (w783:dbl)
                        n3999 = local read "Sampling rate"() -> (w777:dbl)
                        n4000 = local read "finite samples"() -> (w778:bool)
                        n4001 = local read "continuous"() -> (w781:bool)
                        n4002 = local read "wavdet"() -> (w782:bool)
                        n4003 = local read "# of frames"() -> (w780:i32)
                        n4004 = local read "maxbufferAI"() -> (w779:i32)
                        n4005 = local read "Override AI buffer"() -> (w775:bool)
                        n4006 = call "2pparameters.vi"("command"="get") -> ("params out"=w792:T12)  [unwired: 1 in]
                        n4007 = Bundle By Name(cluster=w792, "type"="X-Y-t movie", "avpp"=w795, "Angle Img"=w794, "Xpixels Img"=w790, "Vx-min Img"=w789, "VX-max Img"=w788, "Ypixels Img"=w786, "Vy-min Img"=w787, "Vy-max Img"=w783, "srate"=w777, "srate Img"=w777, "finite"=w778, "cont"=w781, "wavdet"=w782, "measpoints"=w780, "maxbufferAI"=w779, "Drawing Mode"=w793, "Vz-reset"=0.0, "AIoverride"=w775) -> (w784:T12)
                        n4008 = call "2pparameters.vi"("Params in"=w784, "command"="set") -> ()  [unwired: 1 out]
                      }
                      frame "X-Y-Z stack" {
                        n4009 = call "2pparameters.vi"("command"="get") -> ("params out"=w799:T12)  [unwired: 1 in]
                        n4010 = Bundle By Name(cluster=w799, "type"="X-Y-Z stack") -> (w797:T12)
                        n4011 = call "2pparameters.vi"("Params in"=w797, "command"="set") -> ()  [unwired: 1 out]
                      }
                      frame "Lifetime (scan)" {
                        n4012 = call "2pparameters.vi"("command"="get") -> ("params out"=w804:T12)  [unwired: 1 in]
                        n4013 = Bundle By Name(cluster=w804, "type"="Lifetime (scan)") -> (w802:T12)
                        n4014 = call "2pparameters.vi"("Params in"=w802, "command"="set") -> ()  [unwired: 1 out]
                      }
                      frame "Lifetime (contour)" {
                        n4015 = local read "Vy-min draw"() -> (w814:dbl)
                        n4016 = local read "Vy-max draw"() -> (w813:dbl)
                        n4017 = local read "Vx-min draw"() -> (w816:dbl)
                        n4018 = local read "Vx-max draw"() -> (w815:dbl)
                        n4019 = local read "xpixels ref"() -> (w812:i32)
                        n4020 = local read "ypixels ref"() -> (w811:i32)
                        n4021 = local read "ROI Type"() -> (w810:u16)
                        n4022 = local read "srateAODOtt"() -> (w821:dbl)
                        n4023 = local read "# of frames"() -> (w826:i32)
                        n4024 = local read "refreshtime"() -> (w818:dbl)
                        n4025 = local read "Pel"() -> (w809:dbl)
                        n4026 = local read "bin"() -> (w824:dbl)
                        n4027 = local read "Override AI buffer"() -> (w807:bool)
                        n4028 = local read "finite samples"() -> (w833:bool)
                        n4029 = local read "srateAODOtt"() -> (w820:dbl)
                        n4030 = local read "srateAODOtt"() -> (w827:dbl)
                        n4031 = local read "continuous"() -> (w832:bool)
                        n4032 = local read "Angle ref"() -> (w817:dbl)
                        n4033 = local read "wavdet"() -> (w834:bool)
                        n4034 = local read "Vx-ref"() -> (w829:dbl)
                        n4035 = local read "Vy-ref"() -> (w831:dbl)
                        n4036 = local read "avpp"() -> (w830:i32)
                        n4037 = call "tt_timeandsamples.vi"("bin"=w824, "refreshtime"=w818, "srateAODOtt"=w821, "tot#ofsamples"=w826) -> ("refreshrate"=w822:dbl, "refreshbuffer"=w823:i32, "timetracecycles"=w828:i32)  [unwired: 5 in]
                        n4038 = local read "bin"() -> (w825:dbl)
                        n4039 = call "2pparameters.vi"("command"="get") -> ("params out"=w837:T12)  [unwired: 1 in]
                        n4040 = Bundle By Name(cluster=w837, "Drawing Mode"=w810, "measpoints"=w826, "tt_cycles"=w828, "refreshbuffer"=w823, "refreshrate"=w822, "Vx-ref"=w829, "Vy-ref"=w831, "srate"=w820, "finite"=w833, "cont"=w832, "wavdet"=w834, "avpp"=w830, "srateAODO"=w827, "bufferAI"=w823, "bin"=w825, "Angle Img"=w817, "Vxminref"=w816, "Vxmaxref"=w815, "Vyminref"=w814, "Vymaxref"=w813, "Xpixels Img"=w812, "Ypixels Img"=w811, "Pel"=w809, "Vz-reset"=0.0, "AIoverride"=w807, "type"="Lifetime (contour)") -> (w835:T12)
                        n4041 = Reciprocal(x=w822) -> (1/x=w819:dbl)
                        n4042 = local write "refreshtime"(w819) -> ()
                        n4043 = call "2pparameters.vi"("Params in"=w835, "command"="set") -> ()  [unwired: 1 out]
                      }
                      frame "X-Y-Z-t movie" {
                      }
                      frame "linescan" {
                      }
                      frame "Timetrace" {
                        n4044 = local read "Vy-min draw"() -> (w847:dbl)
                        n4045 = local read "Vy-max draw"() -> (w846:dbl)
                        n4046 = local read "Vx-min draw"() -> (w849:dbl)
                        n4047 = local read "Vx-max draw"() -> (w848:dbl)
                        n4048 = local read "xpixels ref"() -> (w845:i32)
                        n4049 = local read "ypixels ref"() -> (w844:i32)
                        n4050 = local read "ROI Type"() -> (w843:u16)
                        n4051 = local read "srateAODOtt"() -> (w854:dbl)
                        n4052 = local read "# of frames"() -> (w859:i32)
                        n4053 = local read "refreshtime"() -> (w851:dbl)
                        n4054 = local read "Pel"() -> (w842:dbl)
                        n4055 = local read "bin"() -> (w857:dbl)
                        n4056 = local read "Override AI buffer"() -> (w840:bool)
                        n4057 = local read "finite samples"() -> (w866:bool)
                        n4058 = local read "srateAODOtt"() -> (w853:dbl)
                        n4059 = local read "srateAODOtt"() -> (w860:dbl)
                        n4060 = local read "continuous"() -> (w865:bool)
                        n4061 = local read "Angle ref"() -> (w850:dbl)
                        n4062 = local read "wavdet"() -> (w867:bool)
                        n4063 = local read "Vx-ref"() -> (w862:dbl)
                        n4064 = local read "Vy-ref"() -> (w864:dbl)
                        n4065 = local read "avpp"() -> (w863:i32)
                        n4066 = call "tt_timeandsamples.vi"("bin"=w857, "refreshtime"=w851, "srateAODOtt"=w854, "tot#ofsamples"=w859) -> ("refreshrate"=w855:dbl, "refreshbuffer"=w856:i32, "timetracecycles"=w861:i32)  [unwired: 5 in]
                        n4067 = local read "bin"() -> (w858:dbl)
                        n4068 = call "2pparameters.vi"("command"="get") -> ("params out"=w870:T12)  [unwired: 1 in]
                        n4069 = Bundle By Name(cluster=w870, "Drawing Mode"=w843, "measpoints"=w859, "tt_cycles"=w861, "refreshbuffer"=w856, "refreshrate"=w855, "Vx-ref"=w862, "Vy-ref"=w864, "srate"=w853, "finite"=w866, "cont"=w865, "wavdet"=w867, "avpp"=w863, "srateAODO"=w860, "bufferAI"=w856, "bin"=w858, "Angle Img"=w850, "Vxminref"=w849, "Vxmaxref"=w848, "Vyminref"=w847, "Vymaxref"=w846, "Xpixels Img"=w845, "Ypixels Img"=w844, "Pel"=w842, "Vz-reset"=0.0, "AIoverride"=w840, "type"="Timetrace") -> (w868:T12)
                        n4070 = Reciprocal(x=w855) -> (1/x=w852:dbl)
                        n4071 = local write "refreshtime"(w852) -> ()
                        n4072 = call "2pparameters.vi"("Params in"=w868, "command"="set") -> ()  [unwired: 1 out]
                      }
                      frame "Lifetime (point)" {
                      }
                    }
                  }
                  frame #1 {
                    w873 = FALSE ("wavdet")
                    n4073 = call "2pparameters.vi"("command"="get") -> ("params out"=w877:T12)  [unwired: 1 in]
                    n4074 = Bundle By Name(cluster=w877, "finite"=w873, "cont"=w873, "wavdet"=TRUE) -> (w874:T12)
                    n4075 = call "2pparameters.vi"("Params in"=w874, "command"="set") -> ()  [unwired: 1 out]
                  }
                  frame #2 {
                    n4076 = local read "DO channels"() -> (w885:u16)
                    n4077 = call "2pparameters.vi"("command"="get") -> ("params out"=w883:T12)  [unwired: 1 in]
                    n4078 = in-place {
                      in-place-border: w885 -> [w890]
                      in-place-border: [w887] -> w880
                      in-place-border: [w886] -> w879
                      n4079 = in-place-cluster #51(w883) -> ("aDO"=w889:u32[])
                      n4080 = call "remove channel from active arrayv2.vi"("line array in"=w889, "line to remove"=w890) -> ("line array out"=w888:u32[], "removal"=w887:bool, "index"=w886:i32)
                      n4081 = in-place-cluster #51("aDO"=w888) -> (w881:T12)
                    }
                    n4082 = local write "remDO"(w880) -> ()
                    n4083 = call "2pparameters.vi"("Params in"=w881, "command"="set") -> ()  [unwired: 1 out]
                  }
                  frame #3 {
                    n4084 = local read "remDO"() -> (w891:bool)
                    n4085 = case shown="True" w891 {
                      frame False {
                      }
                      frame True {
                        n4086 = call "Used AO lines.vi"() -> ("used AO names"=w895:string[], "used AO lines"=w897:tag[])  [unwired: 2 in]
                        n4087 = local write "Analog Used Lines"(w897) -> ()
                        n4088 = local write "Analog Used Names"(w895) -> ()
                        n4089 = call "Used DO lines.vi"() -> ("used DO names"=w893:string[], "used DO lines"=w892:tag[])  [unwired: 2 in]
                        n4090 = control-ref of="Analog Lines Plot"() -> (w896:refnum<vi>)
